vi "ConfigTimeDialog.vi"() -> (0 "Image Folder out":path, 1 "Interval out":dbl format="%<%H:%M:%S>t", 2 "Prefix out":string, 3 "Total out":dbl format="%<%H:%M:%S>t", 5 "Config File Path":path)   [LabVIEW 2018, in "Config.lvlib"]
uses:
  Config.lvlib
panel:
  in  "Finished":bool
  out "Correctness":bool
  in  "Program File Storage":path
  in  "Image Output Folder":path
  in  "File Prefix (\"YYMMDD_HH_mm_SS_\"PREFIX\".tif)":string="Testtest"
  in  "Interval between two Loop Cycles":dbl=900.0 format="%<%H:%M:%S>t"
  in  "Total Acquisition Time":dbl=86400.0 format="%<%H:%M:%S>t"
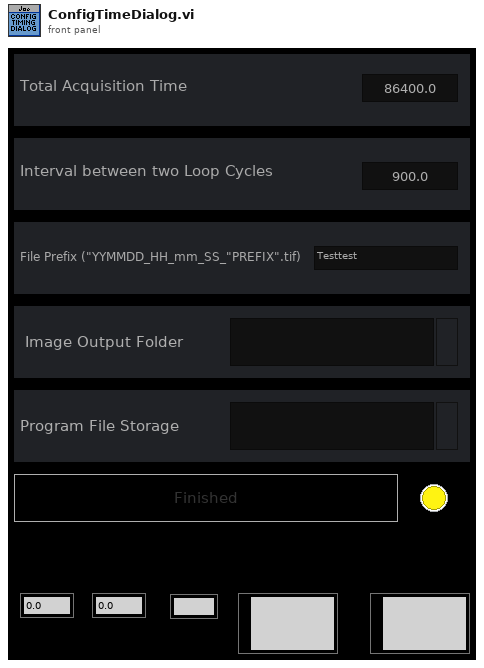
[diagram p1: front panel]
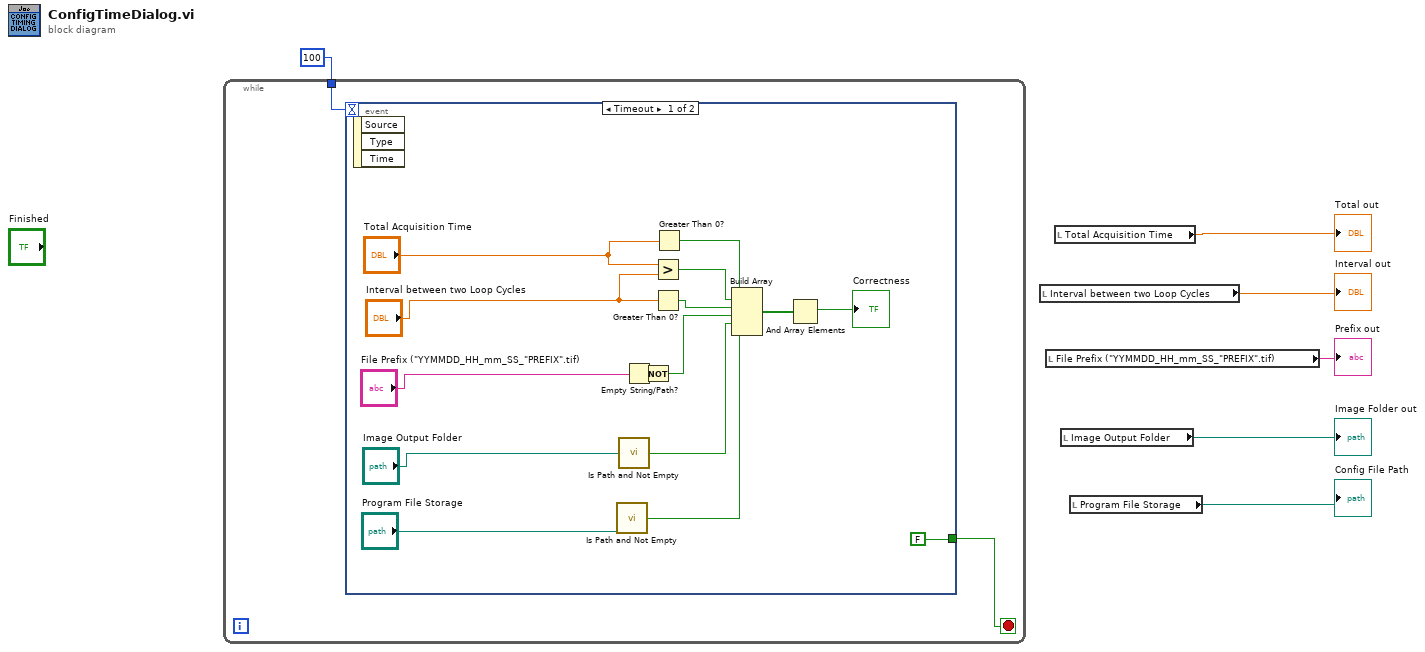
[diagram p0: block diagram]
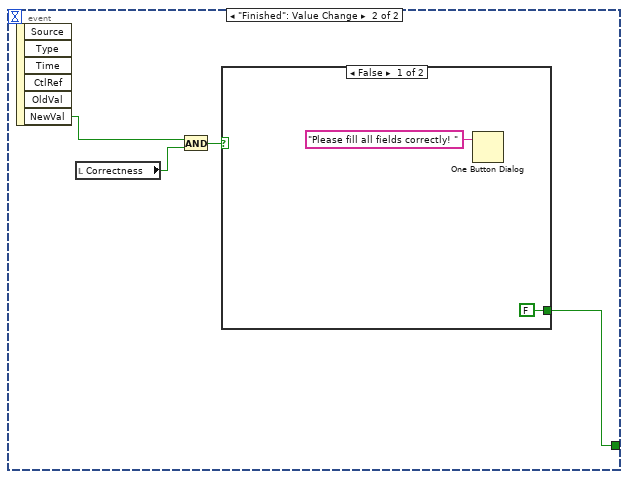
[diagram p2: hidden frame]
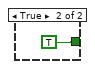
[diagram p3: hidden frame]
diagram:
  n1 = while {
    tunnel: 100 -> [w8]
    stop <- w7 stop-if-true
    n2 = event shown="[0] Timeout" {
      selector: _ -> [_ _]
      dyn-events: _ -> [_ _]
      timeout: w8 -> [_ _]
      tunnel: [FALSE w25] -> w7
      event Timeout {
        n3 = event-data() -> ()  [unwired: 1 in, 3 out]
        n4 = call <vilib>:"Is Path and Not Empty.vi"("path"="Program File Storage") -> ("Is Path and Not Empty?"=w18:bool)  [unwired: 4 in]
        n5 = call <vilib>:"Is Path and Not Empty.vi"("path"="Image Output Folder") -> ("Is Path and Not Empty?"=w19:bool)  [unwired: 4 in]
        n6 = Empty String/Path?(string/path="File Prefix (\"YYMMDD_HH_mm_SS_\"PREFIX\".tif)") -> (empty?=w20:bool)
        n7 = Not(x=w20) -> (.not. x?=w9:bool)
        n8 = Greater?(x="Total Acquisition Time", y="Interval between two Loop Cycles") -> (0:w22:bool)
        n9 = Greater Than 0?(x="Interval between two Loop Cycles") -> (x > 0?=w21:bool)
        n10 = Greater Than 0?(x="Total Acquisition Time") -> (x > 0?=w23:bool)
        n11 = Build Array(w23, w22, w21, w9, w19, w18) -> (w17:bool[])
        n12 = And Array Elements(Boolean array=w17) -> (logical AND=→"Correctness":bool)
      }
      event "Finished": Value Change {
        n13 = event-data() -> ("NewVal"=w26:bool)  [unwired: 1 in, 5 out]
        n14 = local read "Correctness"() -> (w27:bool)
        n15 = And(x=w26, y=w27) -> (x .and. y?=w24:bool)
        n16 = case shown="False" w24 {
          tunnel: [FALSE TRUE] -> w25
          frame False {
            n17 = One Button Dialog(message="Please fill all fields correctly! ") -> ()  [unwired: 1 in, 1 out]
          }
          frame True {
          }
        }
      }
    }
  }
  n18 = local read "Interval between two Loop Cycles"() -> (→"Interval out":dbl)
  n19 = local read "File Prefix (\"YYMMDD_HH_mm_SS_\"PREFIX\".tif)"() -> (→"Prefix out":string)
  n20 = local read "Total Acquisition Time"() -> (→"Total out":dbl)
  n21 = local read "Image Output Folder"() -> (→"Image Folder out":path)
  n22 = local read "Program File Storage"() -> (→"Config File Path":path)
